vi "RP Read RX FIFO Fast.vi"   [LabVIEW 2015]
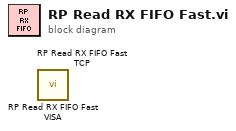
[diagram p0: block diagram]
diagram:
  n1 = call "RP Read RX FIFO Fast VISA.vi"() -> ()  [unwired: 9 in, 3 out]
  n2 = call "RP Read RX FIFO Fast TCP.vi"() -> ()  [unwired: 9 in, 3 out]
